vi "Motion Profile Tester-Speed Target.vi"() -> ()   [LabVIEW 2015]
uses:
  <vilib>/Rock Robotics/WPI/CAN/TalonSRX/WPI_CANTalonSRX_APIControlMode.ctl
  <vilib>/Rock Robotics/WPI/CAN/TalonSRX/WPI_CANTalonSRX_APIFeedbackSelect.ctl
  <vilib>/Rock Robotics/WPI/CAN/TalonSRX/WPI_CANTalonSRX_BrakeOverride.ctl
  OnButton/OnButtonSingle.vi
  <vilib>/Rock Robotics/WPI/MotorControl/WPI_MotorControlOpenCANTalonSRX.vi
panel:
  in  "Max Acceleration (rotations/sec^2)":dbl
  in  "Max Jerk (rotations/sec^3)":dbl
  in  "Speed Target":dbl
  in  "Motion Profile Control Frame Rate":dbl
  in  "Mode":T1(ring)
  in  "Generate, Load, and Run Profile":bool
  in  "Run Profile":bool
  in  "Generate Profile and Clear Points":bool
  in  "Abort":bool
  in  "Run at 100% Power and Graph":bool
  out "Generated Profile":cluster{dbl[], dbl[]}[](graph)
  out "Applied Throttle while Running Profile":cluster{dbl[], dbl[]}(graph)
  out "Motor values while Running Profile":cluster{dbl[], dbl[]}[](graph)
  # "Try to make velocity line slightly below actual motor velocity at 100% power"
  # "If applied throttle exceeds about .95 at any point in the execution of the profile either max  acceleration or jerk must be lowered. If it goes below .8 except at the very beginning or end either max acceleration or jerk  should be increased. (These numbers are for profiles which are supposed to be completed as quickly as possible. In contexts where the priority is on other things such as reducing the amount of force or jerk acting on a gearbox other metrics must be used.)"
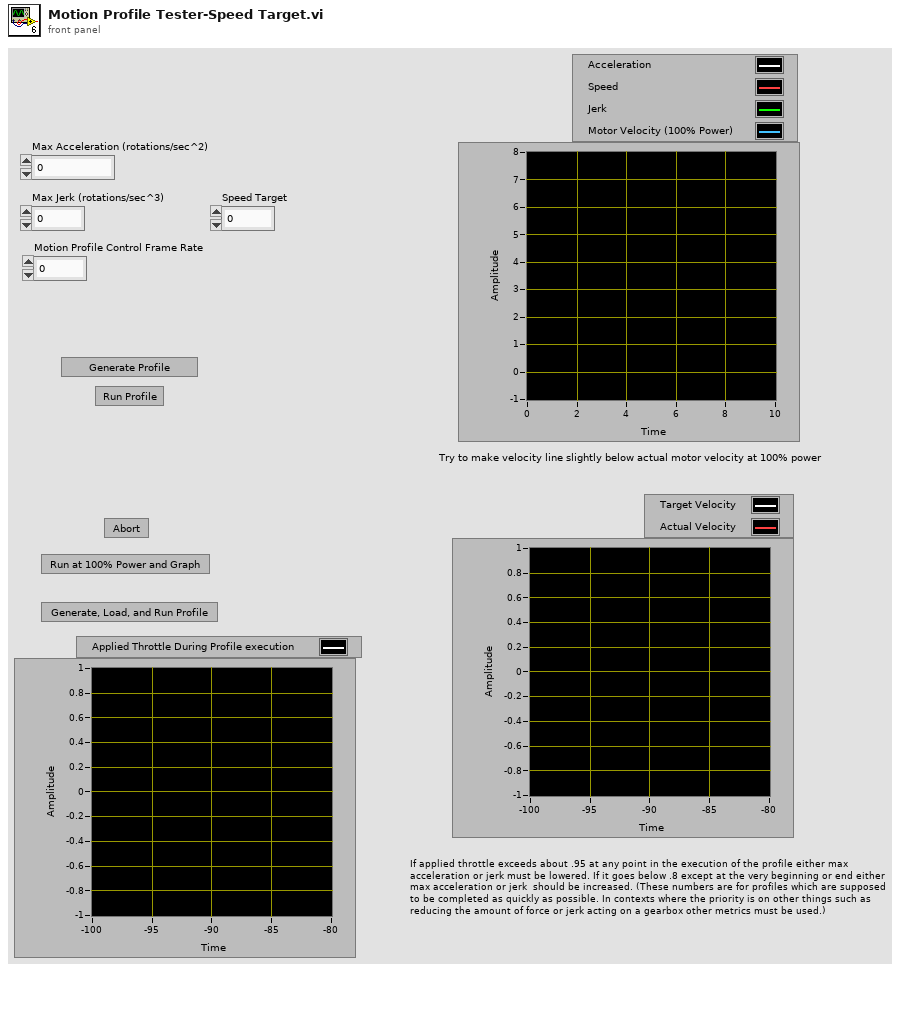
[diagram p1: front panel]
types:
  T1 = enum16{"Nothing", "Generate Profile", "Run Profile", "Run at 100% power and log"}
  T2 = typedef "WPI_CANTalonSRX_BrakeOverride.ctl" = enum8{"No Override", "Override to Coast", "Override to Brake"}
  T3 = typedef "WPI_CANTalonSRX_APIFeedbackSelect.ctl" = enum16{"Digital Quadrature Encoder", "Analog Potentiometer", "Analog Encoder", "Count on Quad-A (Rising-Edge)", "Count on Quad-A (Falling-Edge)", "CTR Magnetic Enc (Absolute)", "CTR Magnetic Enc (Relative)", "Pulse Width"}
  T4 = typedef "WPI_CANTalonSRX_APIControlMode.ctl" = enum8{"Percent VBus", "Speed", "Position", "Slave", "Unchanged / Invalid", "Voltage Compensation", "Current", "Motion Profile"}
  T5 = typedef "WPI_MotorControlDeviceRef.ctl" = cluster{"DeviceStatus":errorcluster, "Type":T6, "PWM":cluster{"PWM Channel":T7, "DeadBand":T8}, "CAN":cluster{"Device Number":u8, "Control Mode":T9, "Semaphore":T10, "Max Vout":dbl, "TalonSRX Control Mode":T4}, "Invert":bool}
  T6 = typedef "WPI_MotorControlType.ctl" = enum16{"PWM", "CAN", "CANTalonSRX"}
  T7 = typedef "FPGA_DIOPWMChannel.ctl" = enum8{"PWM 0", "PWM 1", "PWM 2", "PWM 3", "PWM 4", "PWM 5", "PWM 6", "PWM 7", "PWM 8", "PWM 9", "PWM MXP 0", "PWM MXP 1", "PWM MXP 2", "PWM MXP 3", "PWM MXP 4", "PWM MXP 5", "PWM MXP 6", "PWM MXP 7", "PWM MXP 8", "PWM MXP 9", "Invalid"}
  T8 = typedef "WPI_PWMDeadband.ctl" = cluster{"Name":string, "maxPositivePwm":i32, "minPositivePwm":i32, "centerPwm":i32, "maxNegativePwm":i32, "minNegativePwm":i32, "angularRange":u16}
  T9 = typedef "WPI_CANJaguar_ControlMode.ctl" = enum8{"Percent VBus", "Current", "Speed", "Position", "Voltage"}
  T10 = typedef "Semaphore RefNum" = refnum<k1>
  T11 = enum16{"Nothing", "Generate Profile", "Run Profile", "Run at 100% power and log"}[]
  T12 = typedef "WPI_CANTalonSRX_GlobalStatus.ctl" = cluster{"Applied Throttle":dbl, "Module Enabled":bool, "CAN Error":errorcluster, "Closed Loop Error":dbl, "Forward Limit Switch Closed":bool, "Reverse Limit Switch Closed":bool, "Sensor Position":dbl, "Sensor Velocity":dbl, "Current":dbl, "Sticky Fault - Over Temp":bool, "Sticky Fault - Under Voltage":bool, "Sticky Fault - Forward Limit":bool, "Sticky Fault - Reverse Limit":bool, "Sticky Fault - Forward Soft Limit":bool, "Sticky Fault - Reverse Soft Limit":bool, "Brake is Enabled":bool, "Encoder Position":dbl, "Encoder Velocity":dbl, "Encoder Index Count":dbl, "Encoder A Pin State":bool, "Encoder B Pin State":bool, "Encoder Index Pin State":bool, "Analog In":dbl, "Analog In Velocity":dbl, "Temperature (C)":dbl, "Battery Voltage":dbl, "Control 5 Is Supported":bool, "Current Profile Slot Select":dbl, "Pos Div 8":bool, "Vel Div 4":bool, "Pulse Width Position":i32, "Pulse Width Velocity":i32, "Pulse Width Rise To Rise (us)":i32, "Pulse Width Rise To Fall (us)":i32, "Mot Prof Active Is Under Run":bool, "Mot Prof Active Has Under Run":bool, "Mot Prof Active Is Last":bool, "Mot Prof Active Velocity Only":bool, "Mot Prof Active Is Valid":bool, "Mot Prof Buffer Is Full":bool, "Mot Prof Active Profile Slot Select":i32, "Mot Prof NextID":i32, "Mot Prof Count":i32, "Mot Prof Active Velocity":dbl, "Mot Prof Active Position":dbl, "Mot Prof Output Enable":i32}
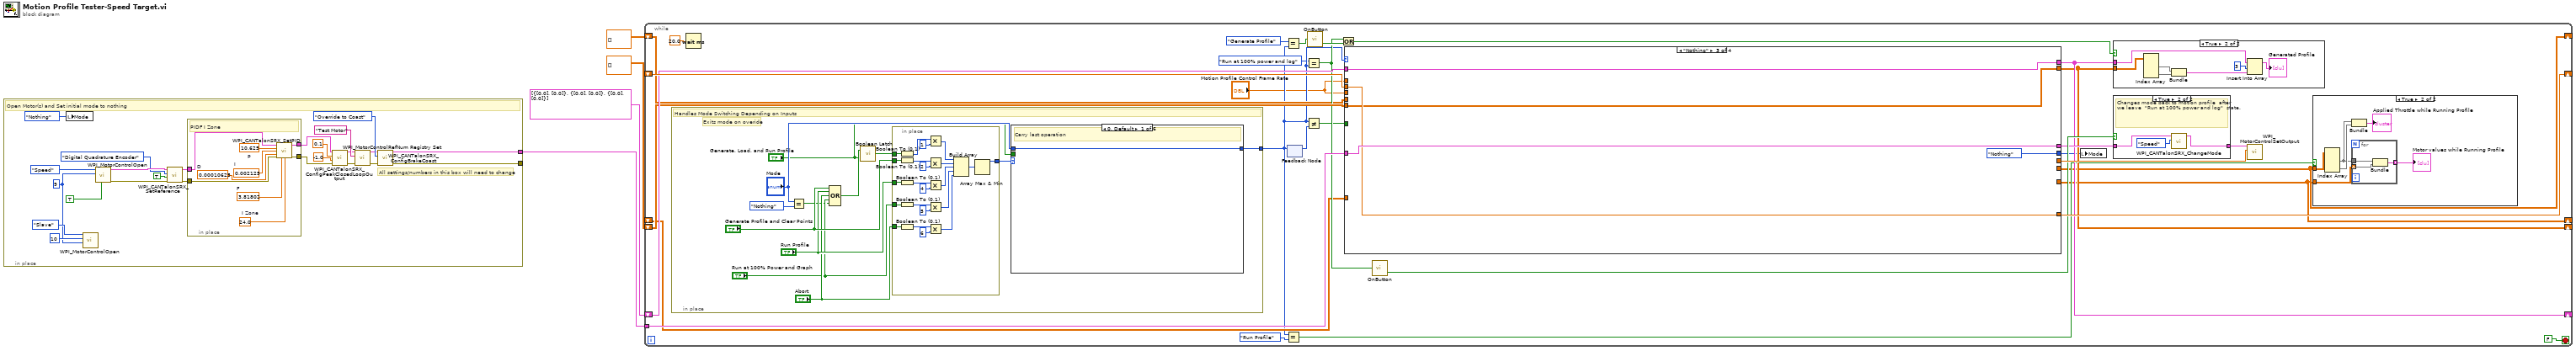
[diagram p0: block diagram]
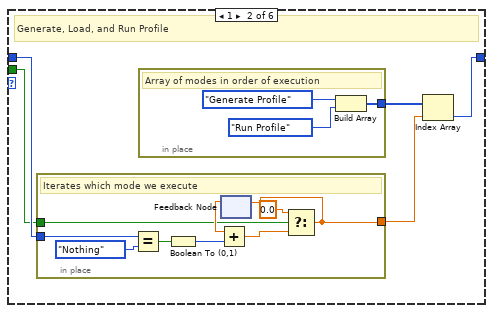
[diagram p5: hidden frame]
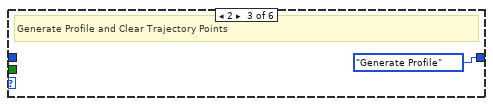
[diagram p6: hidden frame]
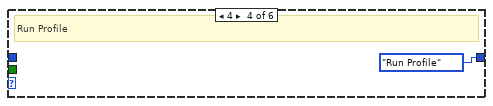
[diagram p7: hidden frame]
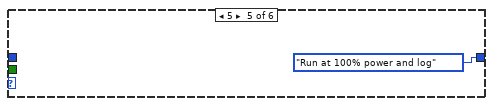
[diagram p8: hidden frame]
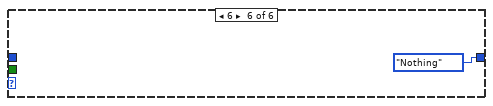
[diagram p9: hidden frame]
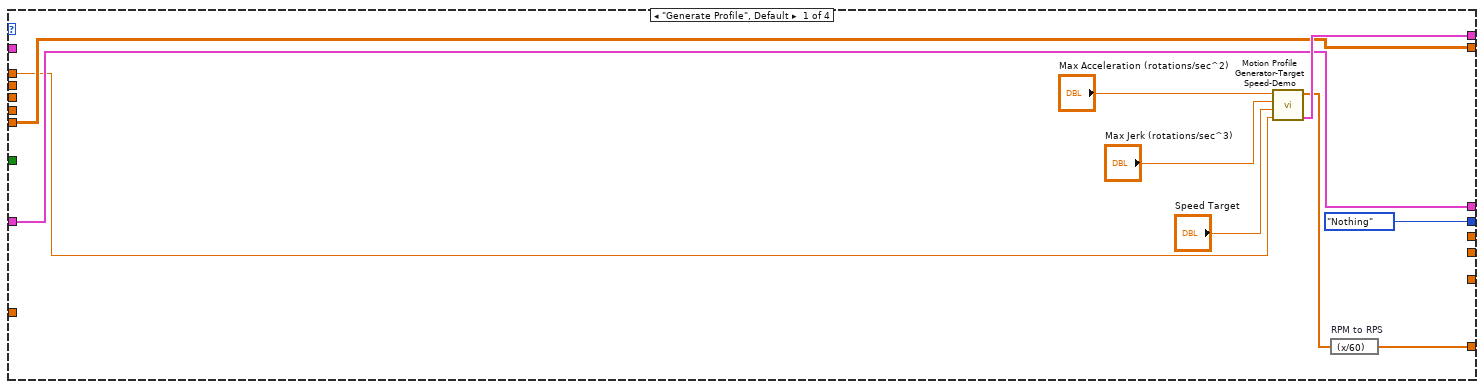
[diagram p10: hidden frame]
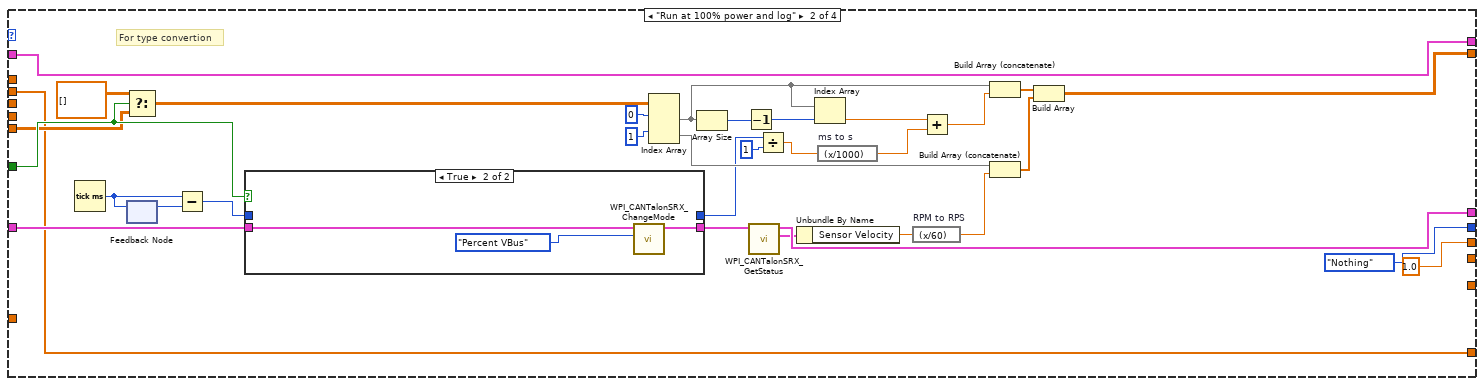
[diagram p11: hidden frame]
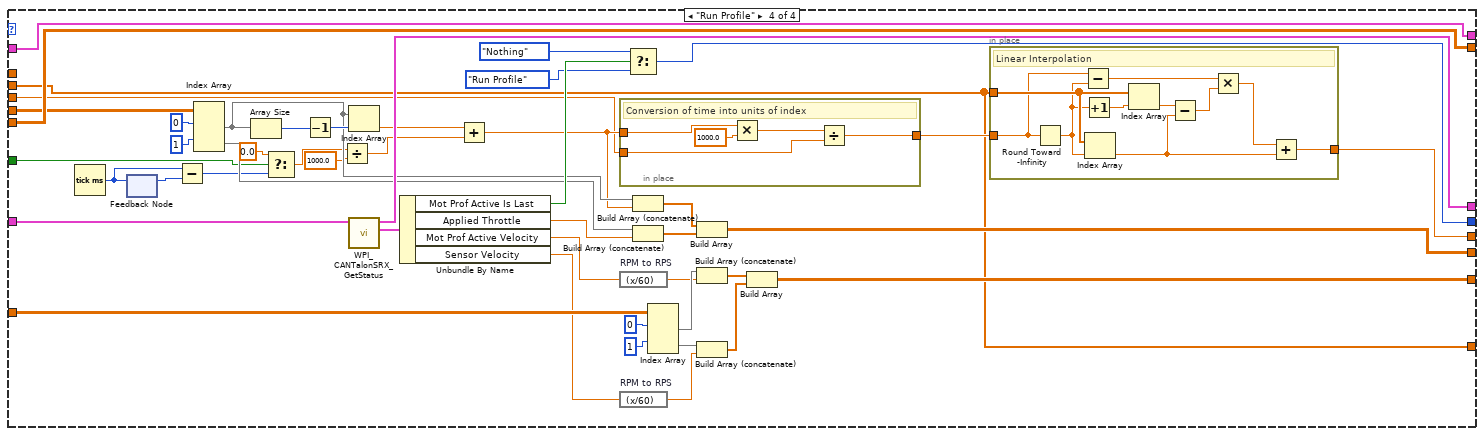
[diagram p13: hidden frame]
diagram:
  n1 = in-place {
    in-place-border: [w19] -> w1
    in-place-border: [w18] -> _
    w25 = u8 9 ("Device Number")
    # "All settings/numbers in this box will need to change"
    # "Open Motor(s) and Set initial mode to nothing"
    n2 = local write "Mode"(T1."Nothing" ("y")) -> ()
    n3 = call-poly <vilib>:"WPI_MotorControlOpen.vi"("Master Device Number"=w25, "Device Number"=u8 10, "Control Mode"=WPI_CANTalonSRX_APIControlMode."Slave") -> ()  [unwired: 7 in, 2 out]
    n4 = call-poly <vilib>:"WPI_MotorControlOpen.vi"("Invert"=TRUE, "Device Number"=w25, "Control Mode"=WPI_CANTalonSRX_APIControlMode."Speed") -> ("error out"=w23:errorcluster, "MotorControlDeviceRef"=w22:T5)  [unwired: 7 in]
    n5 = call <vilib>:"WPI_CANTalonSRX_SetReference.vi"("error in (no error)"=w23, "Reverse Feedback Sensor"=TRUE, "Feedback Reference"=WPI_CANTalonSRX_APIFeedbackSelect."Digital Quadrature Encoder", "CAN Talon SRX Ref"=w22) -> ("error out"=w15:errorcluster, "CAN Talon SRX Ref"=w16:T5)  [unwired: 6 in]
    n6 = in-place {
      in-place-border: [w37] -> w11
      in-place-border: [w36] -> w7
      in-place-border: w16 -> [w35]
      in-place-border: w15 -> [w34]
      w29 = 3.81802  # F
      w30 = 24.0  # I Zone
      w31 = 0.00010625  # D
      w32 = 0.002125  # I
      w33 = 10.625  # P
      # "PIDF I Zone"
      n7 = call <vilib>:"WPI_CANTalonSRX_SetPID.vi"("CAN Talon SRX Ref"=w35, "P"=w33, "I"=w32, "D"=w31, "error in (no error)"=w34, "F"=w29, "I Zone"=w30) -> ("CAN Talon SRX Ref"=w37:T5, "error out"=w36:errorcluster)  [unwired: 7 in]
    }
    n8 = call <vilib>:"WPI_CANTalonSRX_ConfigPeakClosedLoopOutput.vi"("error in (no error)"=w7, "Reverse Peak Output"=-1.0, "Forward Peak Output"=0.1, "CAN Talon SRX Ref"=w11) -> ("error out"=w6:errorcluster, "CAN Talon SRX Ref"=w10:T5)  [unwired: 6 in]
    n9 = call <vilib>:"WPI_MotorControlRefNum Registry Set.vi"("error in (no error)"=w6, "refnum name"="Test Motor", "MotorControlDevRef"=w10) -> ("error out"=w12:errorcluster, "MotorControlDevRef"=w14:T5)  [unwired: 7 in]
    n10 = call <vilib>:"WPI_CANTalonSRX_ConfigBrakeCoast.vi"("error in (no error)"=w12, "Brake / Coast Mode"=WPI_CANTalonSRX_BrakeOverride."Override to Coast", "CAN Talon SRX Ref"=w14) -> ("error out"=w18:errorcluster, "CAN Talon SRX Ref"=w19:T5)  [unwired: 7 in]
  }
  n11 = while {
    tunnel: w1 -> [w67]
    shift-right: [w66] -> _
    shift-left: _ -> [w64]
    shift-right: [w56] -> _
    shift-left: cluster{dbl[], dbl[]}[] [{[0.0], [0.0]}, {[0.0], [0.0]}, {[0.0], [0.0]}] ("XY Graph") -> [w58]
    shift-right: [w55] -> _
    shift-left: dbl[][] [] -> [w57]
    shift-right: [w48] -> _
    shift-left: dbl[][] [] -> [w50]
    shift-right: [w46] -> _
    shift-left: _ -> [w47]
    stop <- FALSE stop-if-true
    n12 = in-place {
      in-place-border: [w99] -> w45
      # "Exits mode on overide"
      # "Handles Mode Switching Depending on Inputs"
      n13 = Equal?(x="Mode", y=T1."Nothing") -> (x = y?=w91:bool)
      n14 = Compound Arithmetic op=OR("Generate Profile and Clear Points", "Run Profile", "Abort", "Run at 100% Power and Graph", w91) -> (w90:bool)
      n15 = call "Boolean Latch.vi"("Input"="Generate, Load, and Run Profile", "Reset"=w90) -> ("Output"=w96:bool)
      n16 = in-place {
        in-place-border: "Generate Profile and Clear Points" -> [w121]
        in-place-border: w96 -> [w117]
        in-place-border: "Run Profile" -> [w115]
        in-place-border: [w113] -> w97
        in-place-border: "Abort" -> [w105]
        in-place-border: "Run at 100% Power and Graph" -> [w102]
        n17 = Boolean To (0,1)(Boolean=w117) -> (0, 1=w111:i16)
        n18 = Boolean To (0,1)(Boolean=w121) -> (0, 1=w120:i16)
        n19 = Boolean To (0,1)(Boolean=w115) -> (0, 1=w112:i16)
        n20 = Boolean To (0,1)(Boolean=w102) -> (0, 1=w101:i16)
        n21 = Boolean To (0,1)(Boolean=w105) -> (0, 1=w104:i16)
        n22 = Multiply(x=w111, y=i16 1) -> (x*y=w108:i16)
        n23 = Multiply(x=w120, y=i16 2) -> (x*y=w107:i16)
        n24 = Multiply(x=w112, y=i16 4) -> (x*y=w106:i16)
        n25 = Multiply(x=w101, y=i16 5) -> (x*y=w100:i16)
        n26 = Multiply(x=w104, y=i16 6) -> (x*y=w103:i16)
        n27 = Build Array(w108, w107, w106, w100, w103) -> (w114:i16[])
        n28 = Array Max & Min(array=w114) -> (max value=w113:i16)  [unwired: 3 out]
      }
      n29 = case shown="0, Default" w97 {
        tunnel: [w122 w123 T1."Generate Profile" ("y") T1."Run Profile" ("y") T1."Run at 100% power and log" ("y") T1."Nothing" ("y")] -> w99
        tunnel: "Mode" -> [w122 w127 _ _ _ _]
        tunnel: "Generate, Load, and Run Profile" -> [_ w126 _ _ _ _]
        frame 0, Default {
          # "Carry last operation"
        }
        frame 1 {
          # "Generate, Load, and Run Profile"
          n30 = in-place {
            in-place-border: w127 -> [w136]
            in-place-border: w126 -> [w132]
            in-place-border: [w129] -> w124
            # "Iterates which mode we execute"
            n31 = Equal?(x=w136, y=T1."Nothing") -> (x = y?=w135:bool)
            n32 = Boolean To (0,1)(Boolean=w135) -> (0, 1=w134:i16)
            n33 = feedback #1() -> (w133:dbl)  [unwired: 1 in]
            n34 = Add(x=w133, y=w134) -> (x+y=w130:dbl)
            n35 = Select(t=0.0, s=w132, f=w130) -> (s? t:f=w129:dbl)
            n36 = feedback-in #1(w129) -> ()
          }
          n37 = in-place {
            in-place-border: [w139] -> w125
            # "Array of modes in order of execution"
            n38 = Build Array(T1."Generate Profile" ("y"), T1."Run Profile" ("y")) -> (w139:T11)
          }
          n39 = Index Array(array=w125, index=w124) -> (element=w123:T1)
        }
        frame 2 {
          # "Generate Profile and Clear Trajectory Points"
        }
        frame 4 {
          # "Run Profile"
        }
        frame 5 {
        }
        frame 6 {
        }
      }
    }
    n40 = Wait (ms)(milliseconds to wait=20.0) -> ()  [unwired: 1 out]
    n41 = Equal?(x=T1."Generate Profile" ("y"), y=w45) -> (x = y?=w54:bool)
    n42 = Equal?(x=w45, y=T1."Run Profile") -> (x = y?=w49:bool)
    n43 = feedback-in #2(w45) -> ()
    n44 = feedback #2() -> (w44:T1)  [unwired: 1 in]
    n45 = Equal?(x=T1."Run at 100% power and log" ("y"), y=w45) -> (x = y?=w51:bool)
    n46 = Not Equal?(x=w45, y=w44) -> (x != y?=w43:bool)
    n47 = call-poly "OnButton.vi"("Input"=w54) -> ("Released"=w53:bool)  [unwired: 1 out]
    n48 = Or(x=w51, y=w53) -> (x .or. y?=w52:bool)
    n49 = case shown="\"Nothing\"" w45 {
      tunnel: w67 -> [w148 w185 w195 w206]
      tunnel: [w146 w156 w194 w196] -> w66
      tunnel: [T1."Nothing" ("y") T1."Nothing" ("y") T1."Nothing" ("y") w239] -> w39
      tunnel: w64 -> [_ w156 w194 w196]
      tunnel: [w148 w182 w195 w241] -> w59
      tunnel: [_ 1.0 _ w198] -> w62
      tunnel: w43 -> [_ w173 _ w218]
      tunnel: [w152 w175 w192 w236] -> w55
      tunnel: [w153 w181 w193 w237] -> w56
      tunnel: w58 -> [_ w181 w193 w237]
      tunnel: w57 -> [w152 w172 w192 w236]
      tunnel: w50 -> [_ _ _ w235]
      tunnel: [_ _ _ w232] -> w48
      tunnel: w47 -> [_ _ _ w227]
      tunnel: [_ _ _ w221] -> w46
      tunnel: "Motion Profile Control Frame Rate" -> [w145 _ _ _]
      tunnel: "Motion Profile Control Frame Rate" -> [_ _ _ w199]
      frame "Generate Profile", Default {
        n50 = call "Motion Profile Generator-Target Speed-Demo.vi"("Motion Profile Control Frame Rate"=w145, "Target Speed"="Speed Target", "Max Jerk (rotations/sec^2)"="Max Jerk (rotations/sec^3)", "Max Acceleration (rotations/sec)"="Max Acceleration (rotations/sec^2)") -> ("XY Graph"=w153:cluster{dbl[], dbl[]}[], "velocity rotations/sec"=w147:dbl[])  [unwired: 4 in, 2 out]
        n51 = expression code="(x/60)" "RPM to RPS"(w147) -> (w146:dbl[])
      }
      frame "Run at 100% power and log" {
        # "For type convertion"
        n52 = Tick Count (ms)() -> (millisecond timer value=w160:u32)
        n53 = Select(t=dbl[][] [], s=w173, f=w172) -> (s? t:f=w170:dbl[][])
        n54 = feedback #3() -> (w159:u32)  [unwired: 1 in]
        n55 = feedback-in #3(w160) -> ()
        n56 = Subtract(x=w160, y=w159) -> (x-y=w158:u32)
        n57 = case shown="True" w173 {
          tunnel: w185 -> [w187 w190]
          tunnel: [w187 w189] -> w183
          tunnel: [w186 _] -> w167
          tunnel: w158 -> [w186 _]
          frame False {
          }
          frame True {
            n58 = call <vilib>:"WPI_CANTalonSRX_ChangeMode.vi"("Control Mode"=WPI_CANTalonSRX_APIControlMode."Percent VBus", "CAN Talon SRX Ref"=w190) -> ("CAN Talon SRX Ref"=w189:T5)  [unwired: 8 in, 1 out]
          }
        }
        n59 = Index Array(array=w170, index (row) #1=0 ("index (row)"), index (row) #2=1 ("index (row)")) -> (element #1=w163:dbl[], element #2=w178:dbl[])  [unwired: 2 in]
        n60 = Array Size(array=w163) -> (size(s)=w164:i32)
        n61 = Decrement(x=w164) -> (x-1=w162:i32)
        n62 = call <vilib>:"WPI_CANTalonSRX_GetStatus.vi"("CAN Talon SRX Ref"=w183) -> ("Talon SRX Status"=w157:T12, "CAN Talon SRX Ref"=w182:T5)  [unwired: 8 in, 1 out]
        n63 = Divide(x=w167, y=u32 1) -> (x/y=w165:dbl)
        n64 = Unbundle By Name(w157) -> ("Sensor Velocity"=w155:dbl)
        n65 = Index Array(array=w163, index=w162) -> (element=w161:dbl)
        n66 = expression code="(x/1000)" "ms to s"(w165) -> (w169:dbl)
        n67 = expression code="(x/60)" "RPM to RPS"(w155) -> (w174:dbl)
        n68 = Add(x=w161, y=w169) -> (x+y=w168:dbl)
        n69 = Build Array (concatenate)(w163, w168) -> (w177:dbl[])
        n70 = Build Array (concatenate)(w178, w174) -> (w176:dbl[])
        n71 = Build Array(w177, w176) -> (w175:dbl[][])
      }
      frame "Nothing" {
      }
      frame "Run Profile" {
        n72 = Tick Count (ms)() -> (millisecond timer value=w220:u32)
        n73 = feedback #4() -> (w219:u32)  [unwired: 1 in]
        n74 = feedback-in #4(w220) -> ()
        n75 = Subtract(x=w220, y=w219) -> (x-y=w216:u32)
        n76 = Index Array(array=w235, index (row) #1=0 ("index (row)"), index (row) #2=1 ("index (row)")) -> (element #1=w213:dbl[], element #2=w233:dbl[])  [unwired: 2 in]
        n77 = Array Size(array=w213) -> (size(s)=w215:i32)
        n78 = Select(t=0.0, s=w218, f=w216) -> (s? t:f=w203:dbl)
        n79 = Decrement(x=w215) -> (x-1=w214:i32)
        n80 = Divide(x=w203, y=1000.0) -> (x/y=w201:dbl)
        n81 = Index Array(array=w213, index=w214) -> (element=w212:dbl)
        n82 = call <vilib>:"WPI_CANTalonSRX_GetStatus.vi"("CAN Talon SRX Ref"=w206) -> ("Talon SRX Status"=w240:T12, "CAN Talon SRX Ref"=w241:T5)  [unwired: 8 in, 1 out]
        n83 = Unbundle By Name(w240) -> ("Mot Prof Active Is Last"=w238:bool, "Applied Throttle"=w234:dbl, "Mot Prof Active Velocity"=w211:dbl, "Sensor Velocity"=w209:dbl)
        n84 = Add(x=w212, y=w201) -> (x+y=w200:dbl)
        n85 = in-place {
          in-place-border: w200 -> [w256]
          in-place-border: w199 -> [w253]
          in-place-border: [w252] -> w197
          # "Conversion of time into units of index"
          n86 = Multiply(x=w256, y=1000.0) -> (x*y=w254:dbl)
          n87 = Divide(x=w254, y=w253) -> (x/y=w252:dbl)
        }
        n88 = expression code="(x/60)" "RPM to RPS"(w211) -> (w210:dbl)
        n89 = expression code="(x/60)" "RPM to RPS"(w209) -> (w208:dbl)
        n90 = Select(t=T1."Nothing" ("y"), s=w238, f=T1."Run Profile" ("y")) -> (s? t:f=w239:T1)
        n91 = Build Array (concatenate)(w213, w200) -> (w231:dbl[])
        n92 = Build Array (concatenate)(w233, w234) -> (w230:dbl[])
        n93 = Index Array(array=w227, index (row) #1=0 ("index (row)"), index (row) #2=1 ("index (row)")) -> (element #1=w229:dbl[], element #2=w207:dbl[])  [unwired: 2 in]
        n94 = Build Array(w231, w230) -> (w232:dbl[][])
        n95 = Build Array (concatenate)(w229, w210) -> (w228:dbl[])
        n96 = Build Array (concatenate)(w207, w208) -> (w222:dbl[])
        n97 = Build Array(w228, w222) -> (w221:dbl[][])
        n98 = in-place {
          in-place-border: w196 -> [w251]
          in-place-border: [w243] -> w198
          in-place-border: w197 -> [w242]
          # "Linear Interpolation"
          n99 = Round Toward -Infinity(1:w242) -> (0:w250:dbl)
          n100 = Subtract(x=w242, y=w250) -> (x-y=w244:dbl)
          n101 = Increment(x=w250) -> (x+1=w249:dbl)
          n102 = Index Array(array=w251, index=w250) -> (element=w246:dbl)
          n103 = Index Array(array=w251, index=w249) -> (element=w248:dbl)
          n104 = Subtract(x=w248, y=w246) -> (x-y=w247:dbl)
          n105 = Multiply(x=w244, y=w247) -> (x*y=w245:dbl)
          n106 = Add(x=w245, y=w246) -> (x+y=w243:dbl)
        }
      }
    }
    n107 = call-poly "OnButton.vi"("Input"=w51) -> ("Released"=w61:bool)  [unwired: 1 out]
    n108 = local write "Mode"(w39) -> ()
    n109 = case shown="True" w52 {
      tunnel: w56 -> [_ w83]
      tunnel: w55 -> [_ w80]
      frame False {
      }
      frame True {
        n110 = Index Array(array=w80) -> (element #1=w79:dbl[], element #2=w78:dbl[])  [unwired: 4 in]
        n111 = Bundle(w79, w78) -> (w77:cluster{dbl[], dbl[]})  [unwired: 1 in]
        n112 = Insert Into Array(array=w83, index=3, new element=w77) -> (→"Generated Profile":cluster{dbl[], dbl[]}[])
      }
    }
    n113 = case shown="True" w61 {
      tunnel: w59 -> [w84 w87]
      tunnel: [w84 w86] -> w60
      frame False {
      }
      frame True {
        # "Changes mode back to motion profile  after we leave  \"Run at 100% power and log\"  state."
        n114 = call <vilib>:"WPI_CANTalonSRX_ChangeMode.vi"("Control Mode"=WPI_CANTalonSRX_APIControlMode."Speed", "CAN Talon SRX Ref"=w87) -> ("CAN Talon SRX Ref"=w86:T5)  [unwired: 8 in, 1 out]
      }
    }
    n115 = call <vilib>:"WPI_MotorControlSetOutput.vi"("Output"=w62, "MotorControlDevRef"=w60) -> ()  [unwired: 7 in, 3 out]
    n116 = case shown="True" w49 {
      tunnel: w48 -> [_ w73]
      tunnel: w46 -> [_ w70]
      frame False {
      }
      frame True {
        n117 = Index Array(array=w73) -> (element #1=w69:dbl[], element #2=w72:dbl[])  [unwired: 4 in]
        n118 = Bundle(w69, w72) -> (→"Applied Throttle while Running Profile":cluster{dbl[], dbl[]})  [unwired: 1 in]
        n119 = for {
          tunnel: w70 -> [w74] mode=indexing
          tunnel: w69 -> [w75]
          tunnel: [w76] -> w68 mode=indexing
          n120 = Bundle(w75, w74) -> (w76:cluster{dbl[], dbl[]})  [unwired: 1 in]
        }
        "Motor values while Running Profile" <- w68
      }
    }
  }
